vi "collectCI_img.vi"() -> (0 "Avg cts/s":dbl, 1 "recorded samples":i32, 2 "wrap":i32)   [LabVIEW 2015]
uses:
  <vilib>/DAQmx/read.llb/DAQmx Read (Counter 1D U32 1Chan NSamp).vi
  <vilib>/DAQmx/miscellaneous.llb/DAQmx Fill In Error Info.vi
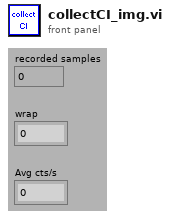
[diagram p1: front panel]
types:
  T1 = typedef "LVRectTypeDef.ctl" = cluster{"Left":i16, "Top":i16, "Right":i16, "Bottom":i16}
  T2 = cluster{"Xpixels":i32, "Vxminref":dbl, "Vxmaxref":dbl, "P":dbl, "Ypixels":i32, "Vyminref":dbl, "Vymaxref":dbl, "srate":sgl, "sAOxy":i32, "timeout":dbl, "type":string, "date":string, "time":string, "Colormap":u16, "Drawing Mode":u16, "Scanning Mode":u16, "square pixels":bool, "square matrix":bool, "Xpixels Img":i32, "Vx-min Img":dbl, "VX-max Img":dbl, "Ypixels Img":i32, "Vy-min Img":dbl, "Vy-max Img ":dbl, "Angle Img":dbl, "autoshutter":bool, "finite":bool, "cont":bool, "wavdet":bool, "measpoints":i32, "avpp":i32, "bufferAO":i32, "bufferAI":i32, "starttick":u32, "waveform":path, "Vx-ref":dbl, "Vy-ref":dbl, "refreshrate":dbl, "refreshbuffer":i32, "tt_cycles":i32, "motorref":refnum<k7>, "mirrorswitch":refnum<k7>, "sample mode":i32, "maxbufferAI":i32, "srateAODO":sgl, "bin":sgl, "Pel":sgl, "Angle draw":dbl, "srate Img":sgl, "ROIimg_plotbounds":T1, "auto OD":bool, "ODfilt":u16, "aAI":i32[], "aCI":i32[], "aAO":u32[], "aDO":u32[], "refwfsize":dbl, "Lifetime":bool, "Vz-Img":dbl, "Vz-ref":dbl, "Vz-reset":dbl, "AIoverride":bool}
  T3 = cluster{"CI":refnum<k21>[], "E_CI":errorcluster[]}
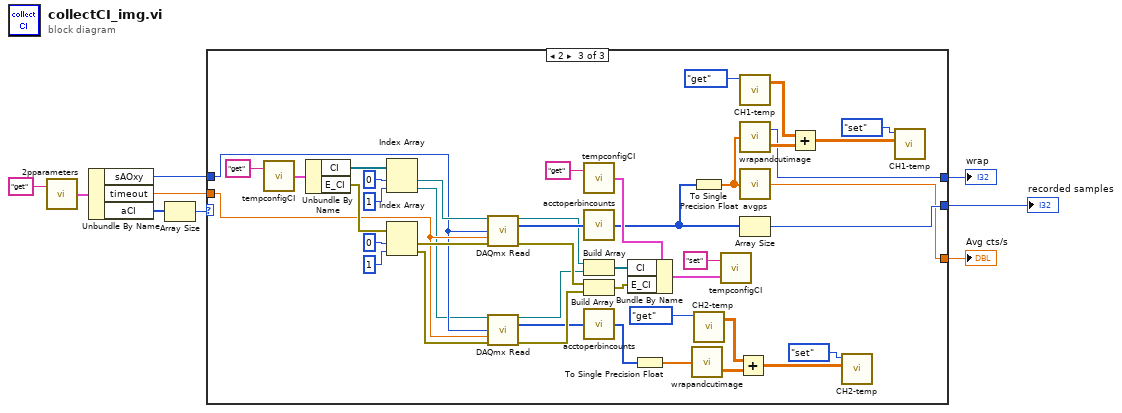
[diagram p0: block diagram]
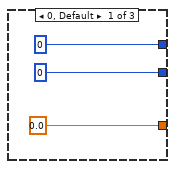
[diagram p2: hidden frame]
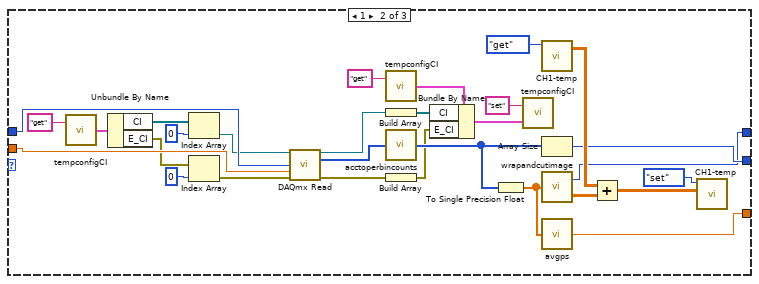
[diagram p3: hidden frame]
diagram:
  n1 = call "2pparameters.vi"("command"="get") -> ("params out"=w9:T2)  [unwired: 1 in]
  n2 = Unbundle By Name(w9) -> ("sAOxy"=w4:i32, "timeout"=w5:dbl, "aCI"=w6:i32[])
  n3 = Array Size(array=w6) -> (size(s)=w7:i32)
  n4 = case shown="2" w7 {
    tunnel: w5 -> [_ w35 w67]
    tunnel: w4 -> [_ w34 w66]
    tunnel: [0 w15 w48] -> w3
    tunnel: [0 ("wrap") w14 w47] -> w2
    tunnel: [0.0 ("Avg cts/s") w13 w46] -> w1
    frame 0, Default {
    }
    frame 1 {
      n5 = call "tempconfigCI.vi"("command"="get") -> ("Temp Config out"=w32:T3)  [unwired: 1 in]
      n6 = Unbundle By Name(w32) -> ("CI"=w30:refnum<k21>[], "E_CI"=w29:errorcluster[])
      n7 = Index Array(array=w30, index=0) -> (element=w27:refnum<k21>)
      n8 = Index Array(array=w29, index=0) -> (element=w26:errorcluster)
      n9 = call-poly <vilib>:"DAQmx Read.vi"("task/channels in"=w27, "number of samples per channel"=w34, "timeout"=w35, "error in"=w26) -> ("task out"=w25:refnum<k21>, "data"=w41:u32[], "error out"=w23:errorcluster)  [unwired: 9 in]
      n10 = call "tempconfigCI.vi"("command"="get") -> ("Temp Config out"=w36:T3)  [unwired: 1 in]
      n11 = Build Array(w25) -> (w24:refnum<k21>[])
      n12 = call "acctoperbincounts.vi"("accumulative counts"=w41) -> ("counts per bin"=w40:u32[])
      n13 = Build Array(w23) -> (w22:errorcluster[])
      n14 = Bundle By Name(cluster=w36, "CI"=w24, "E_CI"=w22) -> (w39:T3)
      n15 = To Single Precision Float(number=w40) -> (single precision float=w16:sgl[])
      n16 = call "tempconfigCI.vi"("Temp Config in"=w39, "command"="set") -> ()  [unwired: 1 out]
      n17 = call "CH1-temp.vi"("command"=enum16{"get", "set", "clear", "add row"}."get") -> ("array out"=w18:sgl[][])  [unwired: 3 in, 1 out]
      n18 = Array Size(array=w40) -> (size(s)=w15:i32)
      n19 = call "wrapandcutimage.vi"("rasterscanned array"=w16) -> ("imagearray"=w19:sgl[][], "wrap"=w14:i32)
      n20 = call "avgps.vi"("data"=w16) -> ("Avg cts/s"=w13:dbl)
      n21 = Add(x=w18, y=w19) -> (x+y=w17:sgl[][])
      n22 = call "CH1-temp.vi"("array in"=w17, "command"=enum16{"get", "set", "clear", "add row"}."set") -> ()  [unwired: 2 in, 2 out]
    }
    frame 2 {
      n23 = call "tempconfigCI.vi"("command"="get") -> ("Temp Config out"=w78:T3)  [unwired: 1 in]
      n24 = Unbundle By Name(w78) -> ("CI"=w69:refnum<k21>[], "E_CI"=w68:errorcluster[])
      n25 = Index Array(array=w69, index #1=0 ("index"), index #2=1 ("index")) -> (element #1=w75:refnum<k21>, element #2=w43:refnum<k21>)
      n26 = Index Array(array=w68, index #1=0 ("index"), index #2=1 ("index")) -> (element #1=w74:errorcluster, element #2=w42:errorcluster)
      n27 = call-poly <vilib>:"DAQmx Read.vi"("task/channels in"=w75, "number of samples per channel"=w66, "timeout"=w67, "error in"=w74) -> ("task out"=w73:refnum<k21>, "data"=w84:u32[], "error out"=w71:errorcluster)  [unwired: 9 in]
      n28 = call-poly <vilib>:"DAQmx Read.vi"("task/channels in"=w43, "number of samples per channel"=w66, "timeout"=w67, "error in"=w42) -> ("task out"=w64:refnum<k21>, "data"=w63:u32[], "error out"=w65:errorcluster)  [unwired: 9 in]
      n29 = call "tempconfigCI.vi"("command"="get") -> ("Temp Config out"=w80:T3)  [unwired: 1 in]
      n30 = call "acctoperbincounts.vi"("accumulative counts"=w84) -> ("counts per bin"=w56:u32[])
      n31 = Build Array(w73, w64) -> (w72:refnum<k21>[])
      n32 = Build Array(w71, w65) -> (w70:errorcluster[])
      n33 = call "acctoperbincounts.vi"("accumulative counts"=w63) -> ("counts per bin"=w49:u32[])
      n34 = Bundle By Name(cluster=w80, "CI"=w72, "E_CI"=w70) -> (w83:T3)
      n35 = To Single Precision Float(number=w49) -> (single precision float=w50:sgl[])
      n36 = call "wrapandcutimage.vi"("rasterscanned array"=w50) -> ("imagearray"=w53:sgl[][])  [unwired: 1 out]
      n37 = To Single Precision Float(number=w56) -> (single precision float=w57:sgl[])
      n38 = call "CH2-temp.vi"("command"=enum16{"get", "set", "clear", "add row"}."get") -> ("array out"=w52:sgl[][])  [unwired: 3 in, 1 out]
      n39 = call "tempconfigCI.vi"("Temp Config in"=w83, "command"="set") -> ()  [unwired: 1 out]
      n40 = Add(x=w52, y=w53) -> (x+y=w51:sgl[][])
      n41 = call "CH1-temp.vi"("command"=enum16{"get", "set", "clear", "add row"}."get") -> ("array out"=w59:sgl[][])  [unwired: 3 in, 1 out]
      n42 = call "wrapandcutimage.vi"("rasterscanned array"=w57) -> ("imagearray"=w60:sgl[][], "wrap"=w47:i32)
      n43 = call "avgps.vi"("data"=w57) -> ("Avg cts/s"=w46:dbl)
      n44 = Array Size(array=w56) -> (size(s)=w48:i32)
      n45 = Add(x=w59, y=w60) -> (x+y=w58:sgl[][])
      n46 = call "CH2-temp.vi"("array in"=w51, "command"=enum16{"get", "set", "clear", "add row"}."set") -> ()  [unwired: 2 in, 2 out]
      n47 = call "CH1-temp.vi"("array in"=w58, "command"=enum16{"get", "set", "clear", "add row"}."set") -> ()  [unwired: 2 in, 2 out]
    }
  }
  "recorded samples" <- w3
  "wrap" <- w2
  "Avg cts/s" <- w1
